vi "SVN_getInfo.vi"(6 "password":string, 7 "username":string, 8 "error in (no error)":errorcluster, 11 "URL":string) -> (0 "error out":errorcluster, 2 "lastChangeDate":string, 3 "revision":i32)   [LabVIEW 2017]
panel:
  out "Command":string
  out "standard output":string
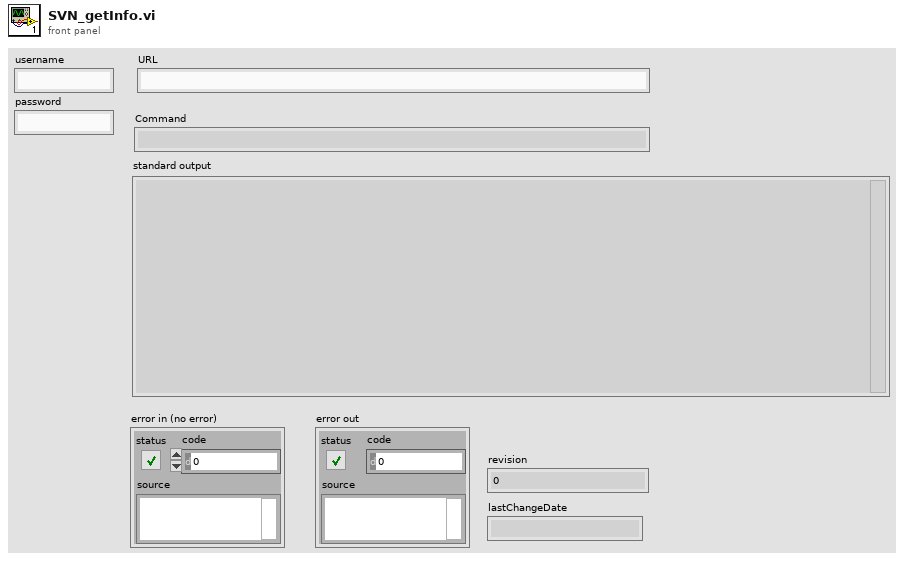
[diagram p1: front panel]
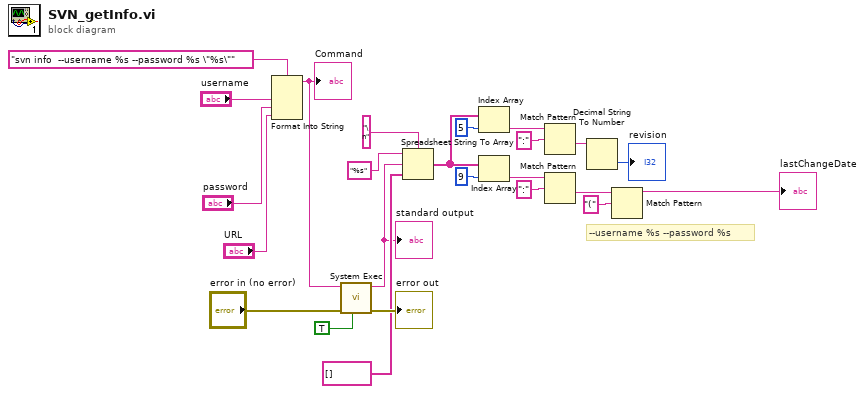
[diagram p0: block diagram]
diagram:
  # "--username %s --password %s"
  n1 = Format Into String(format string="svn info  --username %s --password %s \"%s\"" ("command line"), "username", "password", "URL") -> (resulting string=w20:string)  [unwired: 2 in, 1 out]
  "Command" <- w20
  n2 = call <vilib>:"System Exec.vi"("run minimized? (F)"=TRUE, "error in (no error)"="error in (no error)", "command line"=w20) -> ("error out"=→"error out":errorcluster, "standard output"=w9:string)  [unwired: 5 in, 2 out]
  "standard output" <- w9
  n3 = Spreadsheet String To Array(delimiter (Tab)="\n", format string="%s", spreadsheet string=w9, array type (2D Dbl)=string[] []) -> (array=w5:string[])
  n4 = Index Array(array=w5, index=5) -> (element=w3:string)
  n5 = Index Array(array=w5, index=9) -> (element=w6:string)
  n6 = Match Pattern(string=w3, regular expression=":") -> (after substring=w8:string)  [unwired: 1 in, 3 out]
  n7 = Match Pattern(string=w6, regular expression=":") -> (after substring=w17:string)  [unwired: 1 in, 3 out]
  n8 = Decimal String To Number(string=w8) -> (number=→"revision":i32)  [unwired: 2 in, 1 out]
  n9 = Match Pattern(string=w17, regular expression="(") -> (before substring=→"lastChangeDate":string)  [unwired: 1 in, 3 out]
